vi "Table Function - Paste from Ext-Clipboard.vi"(7 "Cut Section from Clipboard":string[][](array[string]), 8 "error in":errorcluster, 9 "Selection Size":T1, 10 "Selection Start":T1, 11 "Text Table In":string[][](array[string])) -> (0 "error out":errorcluster, 3 "Text Table Out":string[][](array[string]))   [LabVIEW 2018]
uses:
  <vilib>/Utility/miscctls.llb/LVRowAndColumnTypeDef.ctl
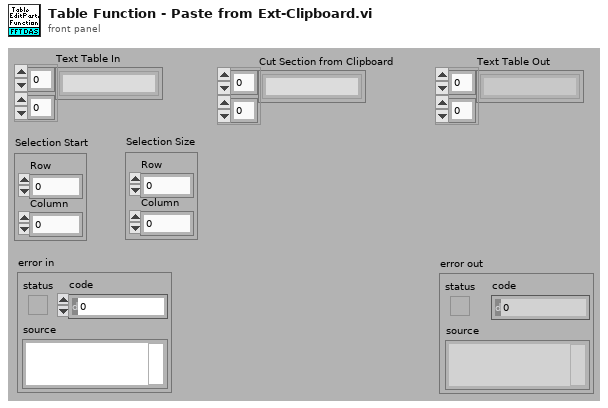
[diagram p1: front panel]
types:
  T1 = typedef "LVRowAndColumnTypeDef.ctl" = cluster{"Row":i32, "Column":i32}
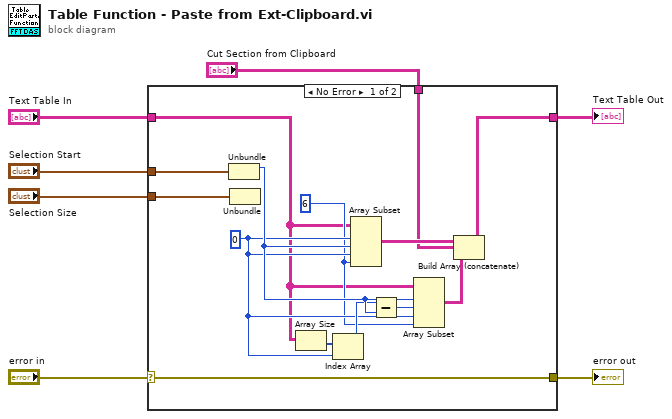
[diagram p0: block diagram]
diagram:
  n1 = case shown="No Error" "error in" {
    selector: "error in" -> [w21 w22]
    tunnel: "Selection Size" -> [w8 _]
    tunnel: "Selection Start" -> [w9 _]
    tunnel: [w11 w23] -> w5
    tunnel: "Text Table In" -> [w12 w23]
    tunnel: [w21 w22] -> w2
    tunnel: "Cut Section from Clipboard" -> [w10 _]
    frame No Error {
      w15 = 6
      w16 = 0
      n2 = Unbundle(w9) -> ("Row"=w20:i32)  [unwired: 1 out]
      n3 = Unbundle(w8) -> ()  [unwired: 2 out]
      n4 = Array Size(array=w12) -> (size(s)=w13:i32[])
      n5 = Index Array(array=w13, index=w16) -> (element=w19:i32)
      n6 = Array Subset(array=w12, index (row)=w16, length (row)=w20, index (col)=w16, length (col)=w15) -> (w14:string[][])
      n7 = Subtract(x=w19, y=w20) -> (x-y=w18:i32)
      n8 = Array Subset(array=w12, index (row)=w20, length (row)=w18, index (col)=w16, length (col)=w15) -> (w17:string[][])
      n9 = Build Array (concatenate)(w14, w10, w17) -> (w11:string[][])
    }
    frame Error {
    }
  }
  "Text Table Out" <- w5
  "error out" <- w2
